vi "save_ttl_time_to_textfile.vi"(4 "Input \nparameters":T2={"Frame rate (ms)"=2000, "Worm strain"="N2", "Time t"=0, "State"=enum."Image acquisition", "Time elapsed"=0.0, "Max_num_runs"=100000, "#TTL"=0, "Time of start TTL"=100000, "ImSub Value"=0, "Time of last TTL"=0, "Number of Columns"=2, "Number of Rows"=2, "# AdjacentTTL"=0, "Sleep deprivation status"="", "Sleep Detection"=FALSE, "# Sleep detections"=0, "Time of first sleep detection"=0, "Time max # adjacent TTL"=0, "Image t-1"=[], "Image t"=[]} {"Number of Rows" items=["1"=1, "2"=2, "3"=3, "4"=4]; "Number of Columns" items=["1"=1, "2"=2, "3"=3, "4"=4]}) -> ()   [LabVIEW 2011]
uses:
  state.ctl
  Action Items.ctl
  Action-Init-Update-Get.ctl
  <vilib>/Utility/file.llb/Write To Spreadsheet File (I64).vi
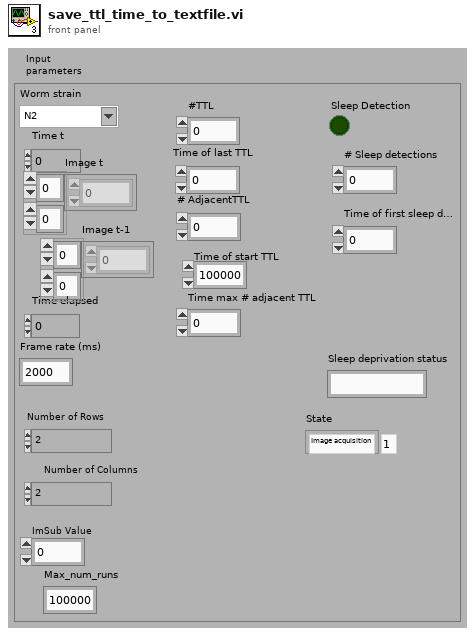
[diagram p1: front panel]
types:
  T1 = typedef "state.ctl" = enum16{"Initialize measurement", "Image acquisition", "Image processing", "Sleep detection", "Control TTL protocol ", "Sleep deprivation", "Update image & exit condition", "Wait "}
  T2 = cluster{"Frame rate (ms)":u32, "Worm strain":string, "Time t":i32, "State":T1, "Time elapsed":dbl, "Max_num_runs":i32, "#TTL":i32, "Time of start TTL":i32, "ImSub Value":i32, "Time of last TTL":i32, "Number of Columns":u32, "Number of Rows":u32, "# AdjacentTTL":i32, "Sleep deprivation status":string, "Sleep Detection":bool, "# Sleep detections":i32, "Time of first sleep detection":i32, "Time max # adjacent TTL":i32, "Image t-1":i32[][], "Image t":i32[][]}
  T3 = typedef "Action-Init-Update-Get.ctl" = enum16{"Initialize", "Update", "Get"}
  T4 = typedef "Action Items.ctl" = enum16{"Initialize", "Get"}
  T5 = cluster{"Path":string, "Filestem":string, "Filestem incl time t":string, "Date":string}
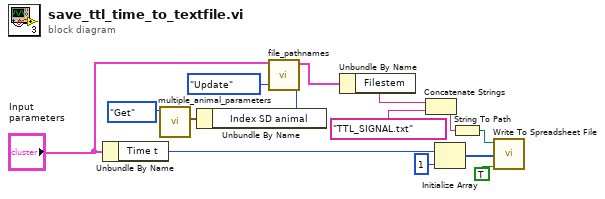
[diagram p0: block diagram]
diagram:
  n1 = Unbundle By Name("Input \nparameters") -> ("Time t"=w8:i32)
  n2 = call "multiple_animal_parameters.vi"("Action"=Action_Items."Get") -> ("Animal\nparameters"=w4:cluster{"# Animals":i32, "Index SD animal":i32})  [unwired: 10 in]
  n3 = Unbundle By Name(w4) -> ("Index SD animal"=w1:i32)
  n4 = call "file_pathnames.vi"("Animal x"=w1, "Action"=Action-Init-Update-Get."Update", "Input \nparameters"="Input \nparameters") -> ("File-path\n-names"=w7:T5)  [unwired: 8 in]
  n5 = Unbundle By Name(w7) -> ("Filestem"=w6:string)
  n6 = Concatenate Strings(w6, "TTL_SIGNAL.txt" ("new file path (Not A Path if cancelled)")) -> (w9:string)
  n7 = Initialize Array(w8, 1 ("Dimension")) -> (w11:i32[])
  n8 = String To Path(string=w9) -> (path=w12:path)
  n9 = call-poly <vilib>:"Write To Spreadsheet File.vi"("append to file? (new file:F)"=TRUE, "1D data"=w11, "file path (dialog if empty)"=w12) -> ()  [unwired: 5 in, 1 out]
